vi "String-Remove trailing zeroes.vi"(11 "String in":string) -> (3 "String out":string)   [LabVIEW 2017]
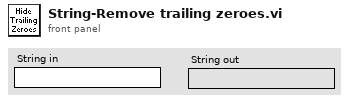
[diagram p1: front panel]
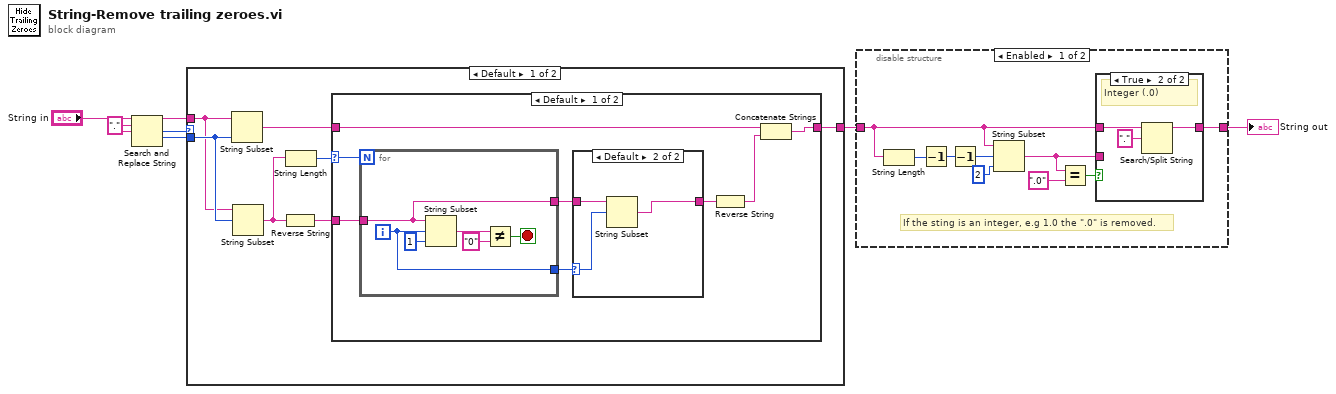
[diagram p0: block diagram]
diagram:
  w6 = "." ("search string")
  n1 = Search and Replace String(input string="String in", search string=w6, replace string=w6) -> (result string=w4:string, number of replacements=w5:i32, offset past replacement=w3:i32)  [unwired: 5 in, 1 out]
  n2 = case shown="Default" w5 {
    tunnel: w4 -> [w13 w34]
    tunnel: [w9 w34] -> w2
    tunnel: w3 -> [w14 _]
    frame Default {
      n3 = String Subset(string=w13, length (rest)=w14) -> (substring=w10:string)  [unwired: 1 in]
      n4 = String Subset(string=w13, offset (0)=w14) -> (substring=w12:string)  [unwired: 1 in]
      n5 = Reverse String(1:w12) -> (0:w8:string)
      n6 = String Length(string=w12) -> (length=w11:i32)
      n7 = case shown="Default" w11 {
        selector: w11 -> [w20 _]
        tunnel: w10 -> [w22 w33]
        tunnel: [w21 w33] -> w9
        tunnel: w8 -> [w19 _]
        frame Default {
          n8 = for {
            N: w20 -> [_]
            tunnel: w19 -> [w27]
            tunnel: [w28] -> w17
            tunnel: [w27] -> w18
            i -> [w28]
            stop <- w29 stop-if-true
            n9 = String Subset(string=w27, offset (0)=w28, length (rest)=1 ("length (rest)")) -> (substring=w31:string)
            n10 = Not Equal?(x=w31, y="0") -> (x != y?=w29:bool)
          }
          n11 = case shown="Default" w17 {
            selector: w17 -> [_ w25]
            tunnel: [w23 w24] -> w16
            tunnel: w18 -> [w23 w26]
            frame 0 {
            }
            frame Default {
              n12 = String Subset(string=w26, offset (0)=w25) -> (substring=w24:string)  [unwired: 1 in]
            }
          }
          n13 = Reverse String(1:w16) -> (0:w15:string)
          n14 = Concatenate Strings(w22, w15) -> (w21:string)
        }
        frame 0 {
        }
      }
    }
    frame 0 {
    }
  }
  n15 = disable-structure shown="Enabled" {
    disable-tunnel: w2 -> [w37 _]
    disable-tunnel: [w36 _] -> w1
    frame Enabled {
      # "If the sting is an integer, e.g 1.0 the \".0\" is removed."
      n16 = String Length(string=w37) -> (length=w43:i32)
      n17 = Decrement(x=w43) -> (x-1=w41:i32)
      n18 = Decrement(x=w41) -> (x-1=w39:i32)
      n19 = String Subset(string=w37, offset (0)=w39, length (rest)=2 ("length (rest)")) -> (substring=w35:string)
      n20 = Equal?(x=w35, y=".0") -> (x = y?=w38:bool)
      n21 = case shown="True" w38 {
        tunnel: w37 -> [w44 w47]
        tunnel: [w44 w45] -> w36
        tunnel: w35 -> [_ _]
        frame False {
        }
        frame True {
          # "Integer (.0)"
          n22 = Search/Split String(string=w47, search string/char (-)=".") -> (substring before match=w45:string)  [unwired: 1 in, 2 out]
        }
      }
    }
    frame Disabled {
    }
  }
  "String out" <- w1
